vi "Current_Path.vi"(1 "Postfix":string="\\", 2 "Dir Or File Name":string="Data") -> (0 "Dir or File In Current Path":path)   [LabVIEW 2009]
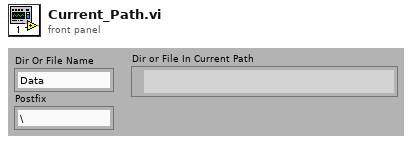
[diagram p1: front panel]
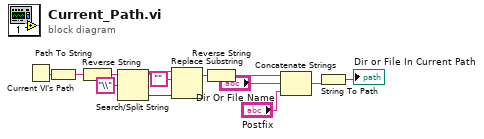
[diagram p0: block diagram]
diagram:
  n1 = Current VI's Path() -> (path=w8:path)
  n2 = Path To String(path=w8) -> (string=w9:string)
  n3 = Reverse String(1:w9) -> (0:w7:string)
  n4 = Search/Split String(string=w7, search string/char (-)="\\") -> (offset of match=w11:i32)  [unwired: 3 out]
  n5 = Replace Substring(2:w11, 4:"", 5:w7) -> (1:w12:string)  [unwired: 2 out]
  n6 = Reverse String(1:w12) -> (0:w5:string)
  n7 = Concatenate Strings(w5, "Dir Or File Name", "Postfix") -> (w2:string)
  n8 = String To Path(string=w2) -> (path=→"Dir or File In Current Path":path)
